vi "Generate Classes Relative Paths File.vi"(6 "Relative Paths File Path":path, 8 "error in (no error)":errorcluster, 9 "Relative Paths File Name":string, 10 "Classes":refnum<class>[](array[class]), 11 "Reference Class":refnum<class>) -> (0 "error out":errorcluster)   [LabVIEW 2023, in "Class Loader.lvlib" / "Class Loader.lvclass"]
uses:
  Class Loader.lvclass
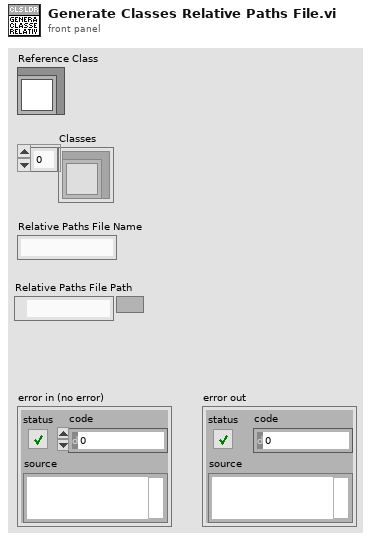
[diagram p1: front panel]
types:
  T1 = enum16{"open", "replace", "create", "open or create", "replace or create", "replace or create with confirmation"}
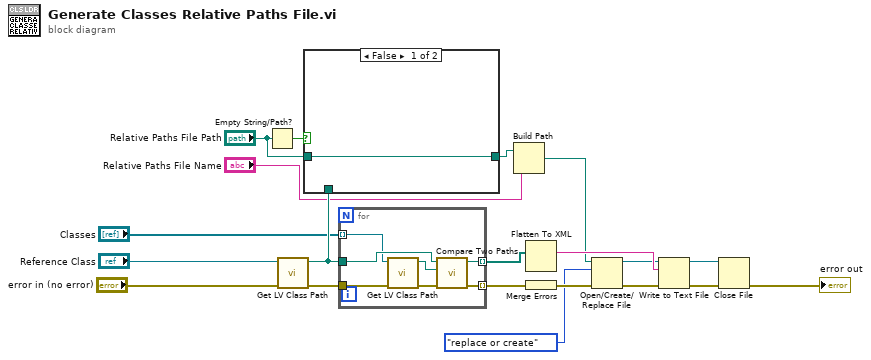
[diagram p0: block diagram]
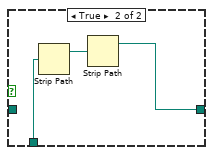
[diagram p2: hidden frame]
diagram:
  n1 = Empty String/Path?(string/path="Relative Paths File Path") -> (empty?=w5:bool)
  n2 = call <vilib>:"Get LV Class Path.vi"("error in (no error)"="error in (no error)", "object"="Reference Class") -> ("error out"=w7:errorcluster, "class path"=w19:path)  [unwired: 8 in]
  n3 = case shown="False" w5 {
    tunnel: w19 -> [_ w24]
    tunnel: "Relative Paths File Path" -> [w21 _]
    tunnel: [w21 w22] -> w2
    frame False {
    }
    frame True {
      n4 = Strip Path(path=w24) -> (stripped path=w23:path)  [unwired: 1 out]
      n5 = Strip Path(path=w23) -> (stripped path=w22:path)  [unwired: 1 out]
    }
  }
  n6 = for {
    tunnel: "Classes" -> [w30] mode=indexing
    tunnel: w19 -> [w31]
    tunnel: w7 -> [w29]
    tunnel: [w25] -> w10 mode=indexing
    tunnel: [w26] -> w9 mode=indexing
    n7 = call <vilib>:"Get LV Class Path.vi"("error in (no error)"=w29, "object"=w30) -> ("error out"=w28:errorcluster, "class path"=w27:path)  [unwired: 8 in]
    n8 = call <vilib>:"Compare Two Paths.vi"("error in (no error)"=w28, "Path 2"=w27, "Path 1"=w31) -> ("error out"=w26:errorcluster, "Relative Path from 1 to 2"=w25:path)  [unwired: 5 in, 2 out]
  }
  n9 = Build Path(base path=w2, name or relative path="Relative Paths File Name") -> (appended path=w1:path)
  n10 = Flatten To XML(6:w10) -> (2:w15:string)
  n11 = Merge Errors(w9) -> (w20:errorcluster)
  n12 = Open/Create/Replace File(file path (use dialog)=w1, error in=w20, operation (0:open)=T1."replace or create") -> (refnum out=w11:refnum<file>, error out=w12:errorcluster)  [unwired: 3 in, 1 out]
  n13 = Write to Text File(file (use dialog)=w11, text=w15, error in=w12) -> (refnum out=w14:refnum<file>, error out=w13:errorcluster)  [unwired: 1 in, 1 out]
  n14 = Close File(refnum=w14, error in=w13) -> (error out=→"error out":errorcluster)  [unwired: 1 out]
